vi "I2C Init Channel.vi"(0 "handle":u32, 5 "Config":T1={"ClockRate"=100000, "LatencyTimer"=1, "Disable 3 phase clocking"=FALSE, "Disable drive only 0"=FALSE} {"ClockRate" items=["I2C_CLOCK_STANDARD_MODE"=100000, "I2C_CLOCK_FAST_MODE"=400000, "I2C_CLOCK_FAST_MODE_PLUS"=1000000, "I2C_CLOCK_HIGH_SPEED_MODE"=3400000]}, 11 "error in (no error)":errorcluster) -> (4 "handle out":u32, 15 "error out":errorcluster)   [LabVIEW 2017, in "libMPSSE.lvlib"]
doc: "FTDI_API FT_STATUS I2C_InitChannel(FT_HANDLE handle, ChannelConfig *config);"
uses:
  libMPSSE.lvlib
  \\Mac\Home/Desktop/libMPSSE-SPI-LabVIEW-master/libMPSSE.dll
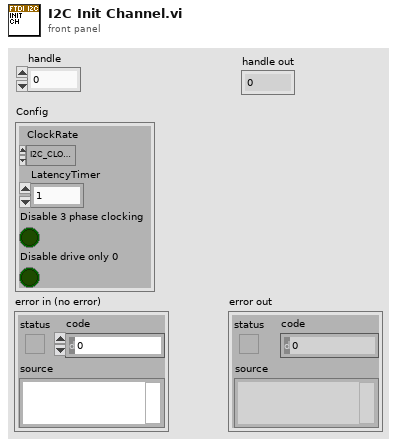
[diagram p1: front panel]
types:
  T1 = cluster{"ClockRate":u32, "LatencyTimer":u8, "Disable 3 phase clocking":bool, "Disable drive only 0":bool}
  T2 = cluster{"ClockRate":u32, "LatencyTimer":u8, "Options":u32}
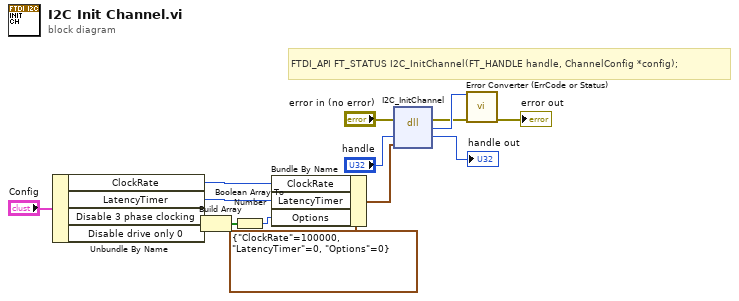
[diagram p0: block diagram]
diagram:
  # "FTDI_API FT_STATUS I2C_InitChannel(FT_HANDLE handle, ChannelConfig *config);"
  n1 = Unbundle By Name("Config") -> ("ClockRate"=w7:u32, "LatencyTimer"=w6:u8, "Disable 3 phase clocking"=w4:bool, "Disable drive only 0"=w5:bool)
  n2 = Build Array(w4, w5) -> (w3:bool[])
  n3 = Boolean Array To Number(Boolean array=w3) -> (number=w2:u32)
  n4 = Bundle By Name(cluster=T2 {"ClockRate"=100000, "LatencyTimer"=0, "Options"=0} ("config"), "ClockRate"=w7, "LatencyTimer"=w6, "Options"=w2) -> (w1:T2)
  n5 = dll-call lib="\\\\Mac\\Home/Desktop/libMPSSE-SPI-LabVIEW-master/libMPSSE.dll" fn="I2C_InitChannel"(error in="error in (no error)", "handle"="handle", "config"=w1) -> (error out=w11:errorcluster, "return type"=w15:u32, "handle"=→"handle out":u32)  [unwired: 3 in, 1 out]
  n6 = call "Error Converter (ErrCode or Status).vi"("error code"=w15, "error in (no error)"=w11) -> ("error out"=→"error out":errorcluster)  [unwired: 13 in]
